vi "Symphony Wavelenght Conv.vi"(4 "Angle Y (deg)":dbl=12.5 format="%#_13g", 6 "Focale":dbl=320.0 format="%#_13g", 7 "PixelArr":ext[](array[numeric]), 8 "error in (no error)":errorcluster, 9 "Angle D(deg)":dbl=21.26 format="%#_13g", 10 "Lambda":dbl, 11 "Grooves(l/mm)":dbl=1800.0 format="%#_13g") -> (0 "error out":errorcluster, 3 "Tableau":dbl[](array[numeric]))   [LabVIEW 2019]
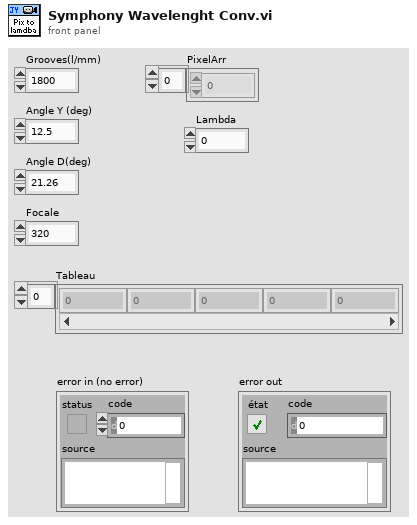
[diagram p1: front panel]
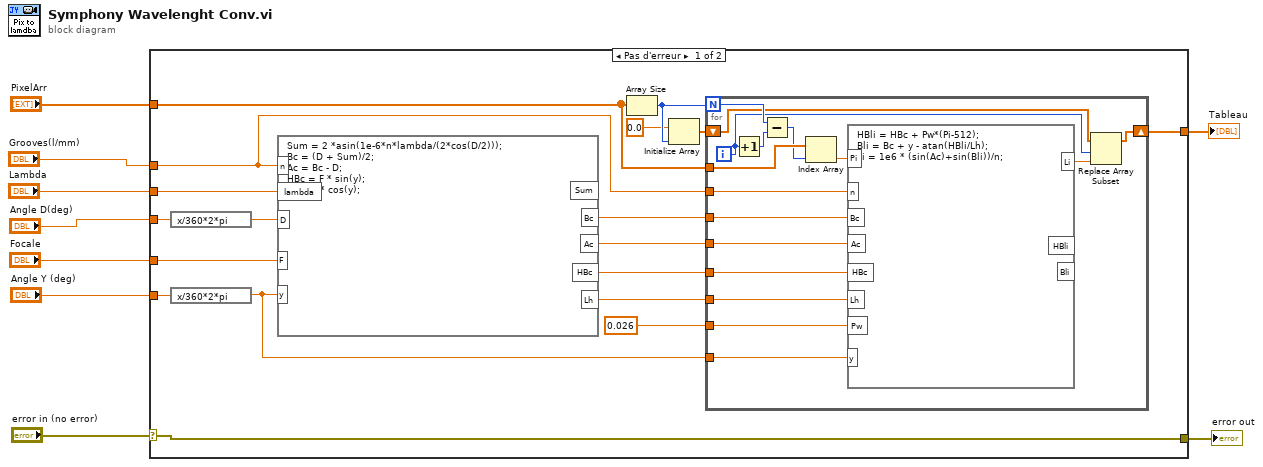
[diagram p0: block diagram]
diagram:
  n1 = case shown="Pas d'erreur" "error in (no error)" {
    selector: "error in (no error)" -> [w22 w44]
    tunnel: "Grooves(l/mm)" -> [w21 _]
    tunnel: "Focale" -> [w27 _]
    tunnel: "Angle Y (deg)" -> [w26 _]
    tunnel: "Angle D(deg)" -> [w24 _]
    tunnel: "Lambda" -> [w23 _]
    tunnel: "PixelArr" -> [w14 _]
    tunnel: [w10 _] -> w3
    tunnel: [w22 w44] -> w1
    frame No Error {
      n2 = expression code="x/360*2*pi"(w24) -> (w25:dbl)
      n3 = expression code="x/360*2*pi"(w26) -> (w18:dbl)
      n4 = formula code="Sum = 2 *asin(1e-6*n*lambda/(2*cos(D/2)));\nBc = (D + Sum)/2;\nAc = Bc - D;\nHBc = F * sin(y);\nLh = F * cos(y);"("n"=w21, "lambda"=w23, "D"=w25, "F"=w27, "y"=w18) -> ("Bc"=w19:dbl, "Ac"=w15:dbl, "HBc"=w16:dbl, "Lh"=w17:dbl)  [unwired: 1 out]
      n5 = Array Size(array=w14) -> (size(s)=w13:i32)
      n6 = Initialize Array(0.0 ("élément"), w13) -> (w12:dbl[])
      n7 = for {
        N: w13 -> [w36]
        tunnel: w21 -> [w43]
        tunnel: 0.026 ("variable en entrée") -> [w42]
        tunnel: w19 -> [w41]
        tunnel: w18 -> [w40]
        tunnel: w17 -> [w39]
        tunnel: w16 -> [w38]
        tunnel: w15 -> [w37]
        tunnel: w14 -> [w34]
        shift-right: [w31] -> w10
        shift-left: w12 -> [w28]
        i -> [w29]
        n8 = Increment(x=w29) -> (x+1=w35:i32)
        n9 = Subtract(x=w36, y=w35) -> (x-y=w32:i32)
        n10 = Index Array(array=w34, index=w32) -> (element=w33:ext)
        n11 = formula code="HBli = HBc + Pw*(Pi-512);\nBli = Bc + y - atan(HBli/Lh);\nLi = 1e6 * (sin(Ac)+sin(Bli))/n;"("n"=w43, "Bc"=w41, "HBc"=w38, "Lh"=w39, "y"=w40, "Pw"=w42, "Pi"=w33, "Ac"=w37) -> ("Li"=w30:dbl)  [unwired: 2 out]
        n12 = Replace Array Subset(array=w28, new element=w30, index=w29) -> (w31:dbl[])
      }
    }
    frame Error {
    }
  }
  "Tableau" <- w3
  "error out" <- w1
